vi "update front panel size.vi"(4 "device ID":refnum<k1>, 6 "screens":T7[](array[typedef]), 8 "error in (no error)":errorcluster, 11 "loop data in":T1) -> (0 "error out":errorcluster, 3 "loop data out":T1)   [LabVIEW 2021, in "TipStripOOPanel.lvlib"]
uses:
  TipStripOOPanel.lvlib
  tipstrip_screens.ctl
  Loop Data Parent.ctl
  <vilib>/IlluminatedG/IG OOPanel/OOPanel/Manager/Manager.lvclass
  Classes/TipPanel/TipPanel.lvclass
  PanelMap.ctl
  PanelMapData.ctl
  Classes/TipPanel/ToPanelUEWrapper.ctl
  Classes/TipPanel/ToPanelUE.ctl
  <vilib>/Futures/Futures/Promise/Promise.lvclass
  refs.ctl
  content size.ctl
  <vilib>/Utility/miscctls.llb/LVRectTypeDef.ctl
  <vilib>/Utility/inputDevices.llb/mouseAcquire.vi
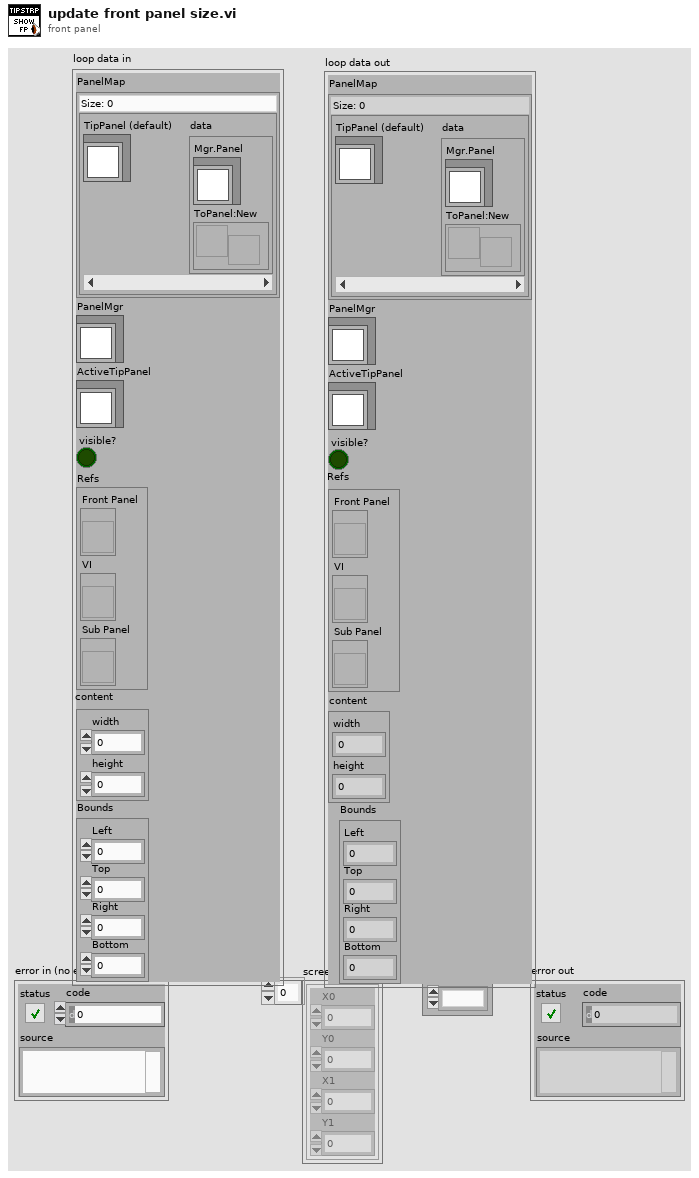
[diagram p1: front panel]
types:
  T1 = typedef "TipStripOOPanel.lvlib/Loop Data Parent.ctl" = cluster{"PanelMap":T2, "PanelMgr":refnum<class "Manager.lvclass">, "ActiveTipPanel":refnum<class "TipPanel.lvclass">, "visible?":bool, "Refs":T4, "content":T5, "Bounds":T6}
  T2 = typedef "TipStripOOPanel.lvlib/PanelMap.ctl" = map{refnum<class "TipPanel.lvclass">, T3}
  T3 = typedef "TipStripOOPanel.lvlib/PanelMapData.ctl" = cluster{"Mgr.Panel":refnum<class "TipPanel.lvclass">, "ToPanel:New":refnum<user-event>}
  T4 = typedef "TipStripOOPanel.lvlib/refs.ctl" = cluster{"Front Panel":refnum<vi>, "VI":refnum<vi>, "Sub Panel":refnum<vi>}
  T5 = typedef "TipStripOOPanel.lvlib/content size.ctl" = cluster{"width":i32, "height":i32}
  T6 = typedef "LVRectTypeDef.ctl" = cluster{"Left":i16, "Top":i16, "Right":i16, "Bottom":i16}
  T7 = typedef "TipStripOOPanel.lvlib/tipstrip_screens.ctl" = cluster{"X0":i32, "Y0":i32, "X1":i32, "Y1":i32}
  T8 = enum32{"Invalid", "Standard", "Closed", "Hidden", "Minimized", "Maximized"}
  T9 = cluster{"Horizontal":i32, "Vertical":i32, "Scrolling":i32}
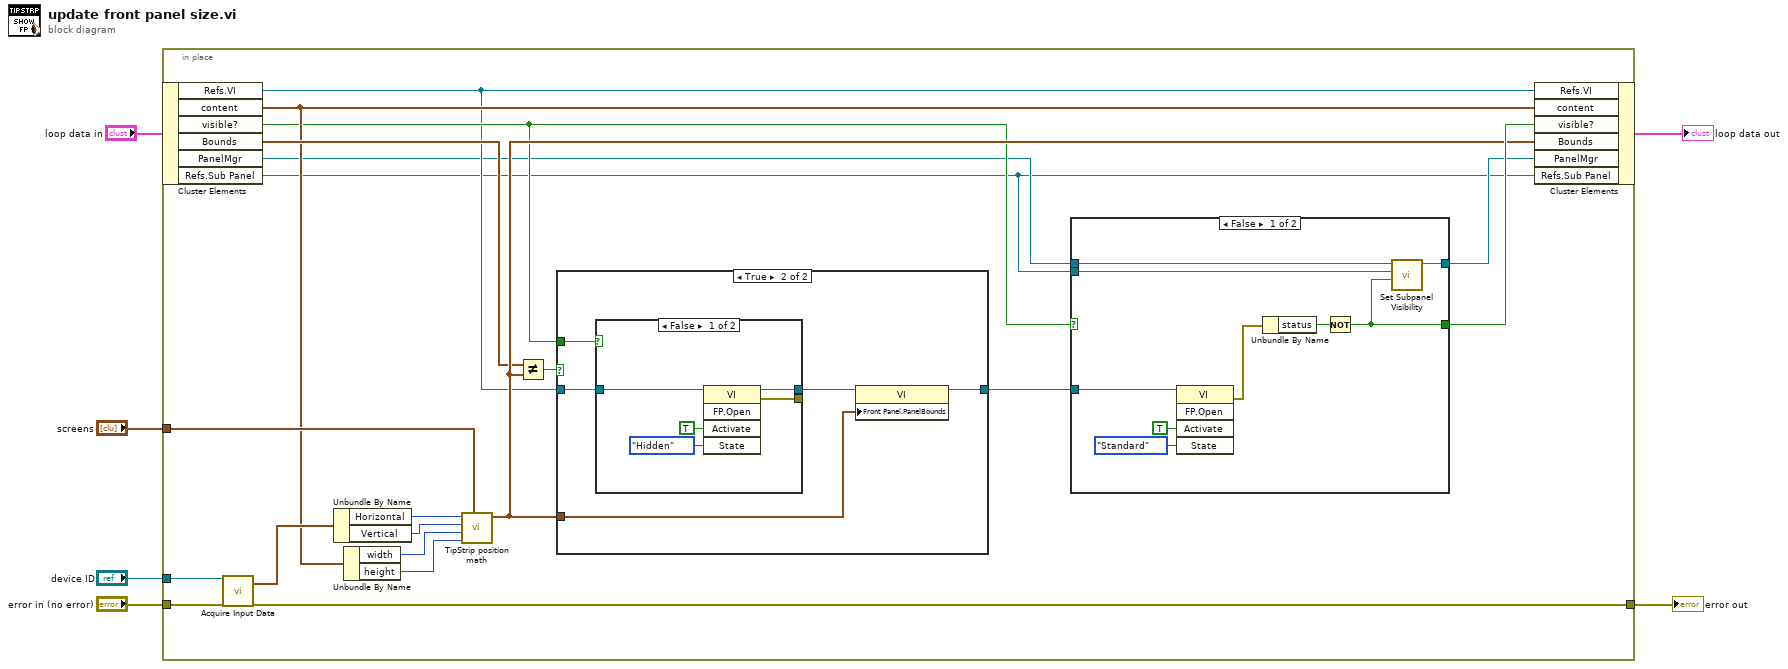
[diagram p0: block diagram]
diagram:
  n1 = in-place {
    in-place-border: "device ID" -> [w22]
    in-place-border: "screens" -> [w20]
    in-place-border: "error in (no error)" -> [w19]
    in-place-border: [w12] -> w3
    n2 = in-place-cluster #1("loop data in") -> ("Refs.VI"=w10:refnum<vi>, "content"=w15:T5, "visible?"=w11:bool, "Bounds"=w16:T6, "PanelMgr"=w9:refnum<class "Manager.lvclass">, "Refs.Sub Panel"=w7:refnum<vi>)
    n3 = call-poly <vilib>:"Acquire Input Data.vi"("device ID"=w22, "error in (no error)"=w19) -> ("axis info"=w26:T9, "error out"=w12:errorcluster)  [unwired: 14 in, 2 out]
    n4 = Unbundle By Name(w26) -> ("Horizontal"=w24:i32, "Vertical"=w23:i32)
    n5 = Unbundle By Name(w15) -> ("width"=w14:i32, "height"=w13:i32)
    n6 = call "TipStrip position math.vi"("screens"=w20, "height"=w13, "width"=w14, "vertical (mouse)"=w23, "horizontal (mouse)"=w24) -> ("Front Panel Window:Panel Bounds"=w17:T6)  [unwired: 6 in]
    n7 = Not Equal?(x=w16, y=w17) -> (x != y?=w18:bool)
    n8 = case shown="True" w18 {
      tunnel: w10 -> [w27 w29]
      tunnel: [w27 w32] -> w25
      tunnel: w17 -> [_ w31]
      tunnel: w11 -> [_ w30]
      frame False {
      }
      frame True {
        n9 = case shown="False" w30 {
          tunnel: w29 -> [w37 w38]
          tunnel: [w34 w38] -> w28
          tunnel: [w33 _] -> _
          frame False {
            n10 = invoke class="VI" method="FP.Open"(reference=w37, "Activate"=TRUE ("Activate?"), "State"=T8."Hidden") -> (reference out=w34:refnum<vi>, error out=w33:errorcluster)  [unwired: 2 in, 3 out]
          }
          frame True {
          }
        }
        n11 = property class="VI"(reference=w28, "Front Panel.PanelBounds"=w31) -> (reference out=w32:refnum<vi>)  [unwired: 1 in, 1 out]
      }
    }
    n12 = case shown="False" w11 {
      selector: w11 -> [_ w49]
      tunnel: w25 -> [w47 _]
      tunnel: [w39 w49] -> w21
      tunnel: w9 -> [w43 w48]
      tunnel: [w42 w48] -> w8
      tunnel: w7 -> [w41 _]
      frame False {
        n13 = invoke class="VI" method="FP.Open"(reference=w47, "Activate"=TRUE ("Activate?"), "State"=T8."Standard") -> (error out=w40:errorcluster)  [unwired: 2 in, 4 out]
        n14 = Unbundle By Name(w40) -> ("status"=w44:bool)
        n15 = Not(x=w44) -> (.not. x?=w39:bool)
        n16 = call <vilib>:"Set Subpanel Visibility.vi"("Visible"=w39, "SubPanel"=w41, "Manager in"=w43) -> ("Manager out"=w42:refnum<class "Manager.lvclass">)  [unwired: 7 in, 1 out]
      }
      frame True {
      }
    }
    n17 = in-place-cluster #1("Refs.VI"=w10, "content"=w15, "visible?"=w21, "Bounds"=w17, "PanelMgr"=w8, "Refs.Sub Panel"=w7) -> (→"loop data out":T1)
  }
  "error out" <- w3
